vi "Untitled 2.vi"() -> ()   [LabVIEW 2020]
panel:
  out "Area":dbl
  in  "Base":dbl
  in  "Altura":dbl
  in  "Slide":dbl(slide) scale=0.0..100.0
  out "Meter":dbl(knob) scale=0.0..100.0
  out "Thermometer":dbl(slide) scale=0.0..100.0
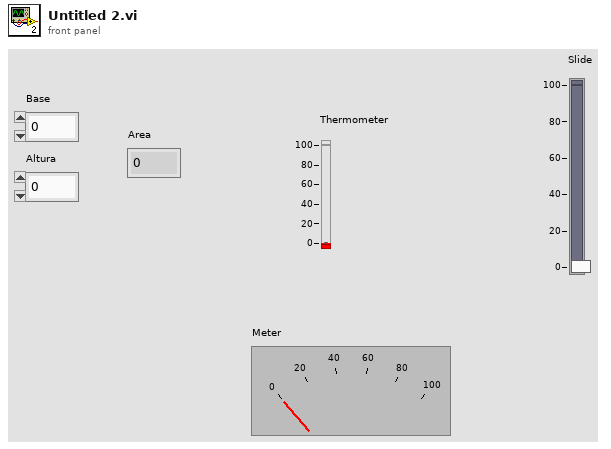
[diagram p1: front panel]
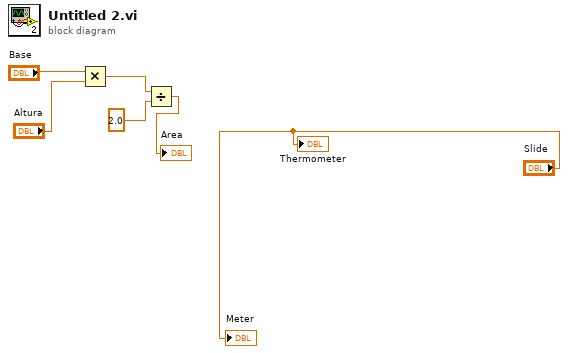
[diagram p0: block diagram]
diagram:
  n1 = Multiply(x="Base", y="Altura") -> (x*y=w1:dbl)
  n2 = Divide(x=w1, y=2.0) -> (x/y=→"Area":dbl)
  "Thermometer" <- "Slide"
  "Meter" <- "Slide"
